vi "设备-tcp侦听配置服务器.vi"() -> ()   [LabVIEW 2013]
panel:
  out "队列中元素数量":i32
  in  "停止按钮":bool
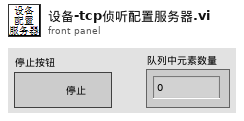
[diagram p1: front panel]
types:
  T1 = cluster{"服务器信息":cluster{"IP":string, "Port":u16}, "账户信息":cluster{"账户可用？":bool, "用户名":string, "密码":string}}
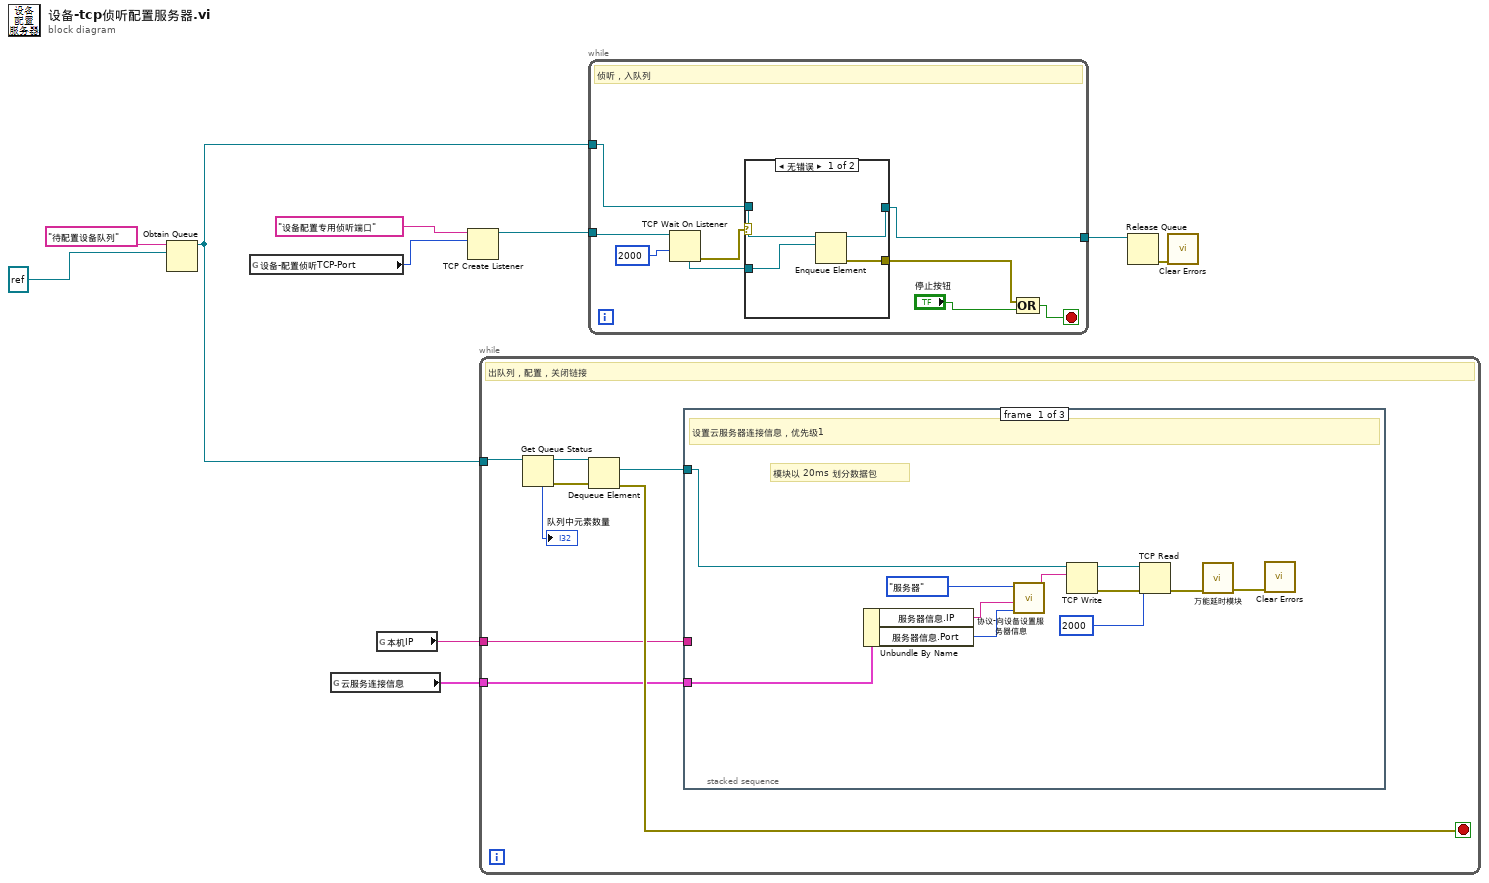
[diagram p0: block diagram]
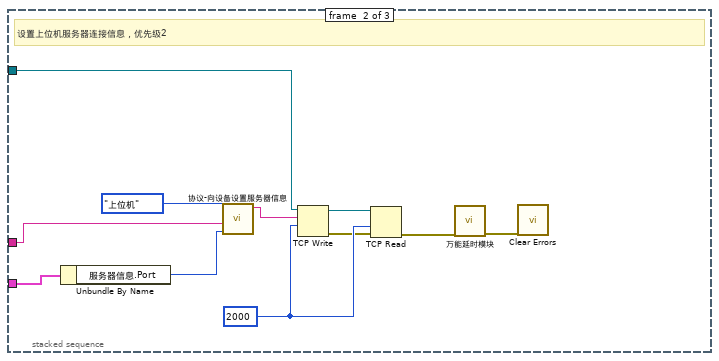
[diagram p2: hidden frame]
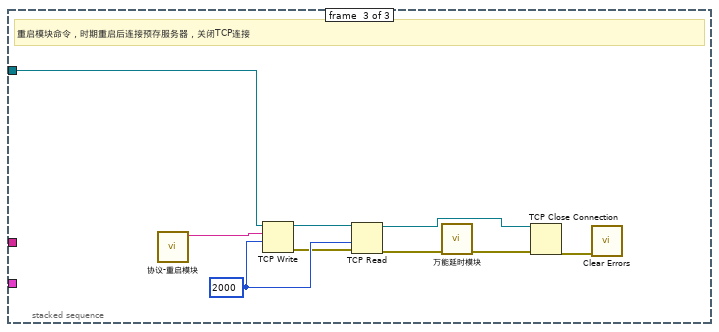
[diagram p3: hidden frame]
diagram:
  n1 = Obtain Queue(name (unnamed)="待配置设备队列" ("名称（未命名）"), element data type=refnum<k5> refnum ("连接ID")) -> (queue out=w6:refnum<queue>)  [unwired: 3 in, 2 out]
  n2 = global read "Client-全局变量.vi" "设备-配置侦听TCP-Port"() -> (w10:u16)
  n3 = global read "Client-全局变量.vi" "云服务连接信息"() -> (w2:T1)
  n4 = global read "Client-全局变量.vi" "本机IP"() -> (w1:string)
  n5 = TCP Create Listener(10:w10, 11:"设备配置专用侦听端口" ("服务名称")) -> (3:w8:refnum<k5>)  [unwired: 3 in, 2 out]
  n6 = while {
    tunnel: w6 -> [w14]
    tunnel: w2 -> [w16]
    tunnel: w1 -> [w15]
    stop <- w18 stop-if-true
    # "出队列，配置，关闭链接"
    n7 = Get Queue Status(queue=w14) -> (queue out=w13:refnum<queue>, error out=w11:errorcluster, # elements in queue=→"队列中元素数量":i32)  [unwired: 2 in, 5 out]
    n8 = Dequeue Element(queue=w13, error in (no error)=w11) -> (element=w17:refnum<k5>, error out=w18:errorcluster)  [unwired: 1 in, 2 out]
    n9 = stacked-sequence {
      tunnel: w17 -> [w29 w35 w48]
      tunnel: w16 -> [w20 w39 _]
      tunnel: w15 -> [_ w38 _]
      frame #0 {
        # "模块以 20ms 划分数据包"
        # "设置云服务器连接信息，优先级1"
        n10 = Unbundle By Name(w20) -> ("服务器信息.IP"=w26:string, "服务器信息.Port"=w25:u16)
        n11 = call "协议-向设备设置服务器信息.vi"("端口"=w25, "IP地址"=w26, "服务器/上位机？"=enum8{"服务器", "上位机"}."服务器") -> ("完整输出"=w28:string)  [unwired: 8 in]
        n12 = TCP Write(connection ID=w29, data in=w28) -> (connection ID out=w22:refnum<k5>, error out=w24:errorcluster)  [unwired: 2 in, 1 out]
        n13 = TCP Read(connection ID=w22, error in (no error)=w24, 9:2000 ("超时毫秒(25000)")) -> (error out=w23:errorcluster)  [unwired: 2 in, 2 out]
        n14 = call "万能延时模块.vi"("错误输入"=w23) -> ("错误输出"=w19:errorcluster)  [unwired: 9 in, 1 out]
        n15 = call <vilib>:"Clear Errors.vi"("error in (no error)"=w19) -> ()  [unwired: 6 in, 1 out]
      }
      frame #1 {
        w34 = 2000 ("超时毫秒(25000)")
        # "设置上位机服务器连接信息，优先级2"
        n16 = Unbundle By Name(w39) -> ("服务器信息.Port"=w37:u16)
        n17 = call "协议-向设备设置服务器信息.vi"("端口"=w37, "IP地址"=w38, "服务器/上位机？"=enum8{"服务器", "上位机"}."上位机") -> ("完整输出"=w36:string)  [unwired: 8 in]
        n18 = TCP Write(connection ID=w35, data in=w36, 9:w34) -> (connection ID out=w32:refnum<k5>, error out=w33:errorcluster)  [unwired: 1 in, 1 out]
        n19 = TCP Read(connection ID=w32, error in (no error)=w33, 9:w34) -> (error out=w31:errorcluster)  [unwired: 2 in, 2 out]
        n20 = call "万能延时模块.vi"("错误输入"=w31) -> ("错误输出"=w30:errorcluster)  [unwired: 9 in, 1 out]
        n21 = call <vilib>:"Clear Errors.vi"("error in (no error)"=w30) -> ()  [unwired: 6 in, 1 out]
      }
      frame #2 {
        w46 = 2000 ("超时毫秒(25000)")
        # "重启模块命令，时期重启后连接预存服务器，关闭TCP连接"
        n22 = call "协议-重启模块.vi"() -> ("完整输出"=w49:string)  [unwired: 11 in]
        n23 = TCP Write(connection ID=w48, data in=w49, 9:w46) -> (connection ID out=w47:refnum<k5>, error out=w45:errorcluster)  [unwired: 1 in, 1 out]
        n24 = TCP Read(connection ID=w47, error in (no error)=w45, 9:w46) -> (connection ID out=w42:refnum<k5>, error out=w44:errorcluster)  [unwired: 2 in, 1 out]
        n25 = call "万能延时模块.vi"("错误输入"=w44) -> ("错误输出"=w43:errorcluster)  [unwired: 9 in, 1 out]
        n26 = TCP Close Connection(connection ID=w42, error in (no error)=w43) -> (error out=w41:errorcluster)  [unwired: 1 in, 1 out]
        n27 = call <vilib>:"Clear Errors.vi"("error in (no error)"=w41) -> ()  [unwired: 6 in, 1 out]
      }
    }
  }
  n28 = while {
    tunnel: w8 -> [w58]
    tunnel: w6 -> [w54]
    tunnel: [w50] -> w4
    stop <- w51 stop-if-true
    # "侦听，入队列"
    n29 = TCP Wait On Listener(9:2000 ("超时毫秒（一直等待:-1）"), 11:w58) -> (0:w56:errorcluster, 4:w55:refnum<k5>)  [unwired: 2 in, 3 out]
    n30 = case shown="无错误" w56 {
      tunnel: w55 -> [w62 _]
      tunnel: w54 -> [w61 w63]
      tunnel: [w60 _] -> w53
      tunnel: [w59 w63] -> w50
      frame No Error {
        n31 = Enqueue Element(queue=w61, element=w62) -> (queue out=w59:refnum<queue>, error out=w60:errorcluster)  [unwired: 2 in, 1 out]
      }
      frame Error {
      }
    }
    n32 = Compound Arithmetic op=OR(w53, "停止按钮") -> (w51:bool)
  }
  n33 = Release Queue(queue=w4) -> (error out=w3:errorcluster)  [unwired: 2 in, 2 out]
  n34 = call <vilib>:"Clear Errors.vi"("error in (no error)"=w3) -> ()  [unwired: 6 in, 1 out]
